vi "WLAN_be_EVM_SA.vi"(5 "Function":T1, 8 "error in":errorcluster, 11 "VISA IN":refnum<visa-resource-name>="IQGIG") -> (0 "error out":errorcluster, 1 "EVM":dbl format="%.0g", 2 "Power":dbl format="%#.3g", 3 "IDN":string)   [LabVIEW 2023, in "LitePoints.lvlib"]
uses:
  LitePoints.lvlib
  CTL/LitePoint_EVM_SA.ctl
  FTDI/JIO/CLC_JIO_FTDI.lvlib
panel:
  out "forREF_PW":string
  out "Response_EVM":string
  out "Response_PW":string
  out "VSA_Ref?":string
  out "VSA?":string
  out "Clean Buffer?":string
  # "IQgig-5G : TCPIP0::192.168.100.254::hislip0::INSTR"
  # "IQxel-MX : TCPIP0::192.168.100.253::hislip0::INSTR"
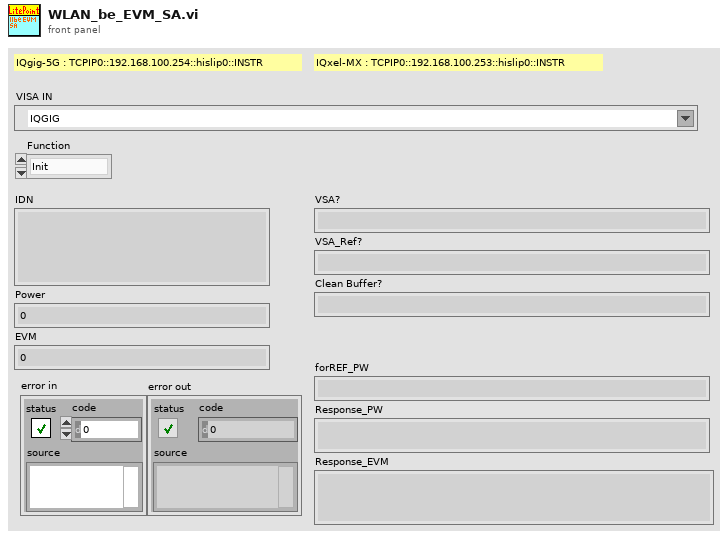
[diagram p1: front panel]
types:
  T1 = typedef "LitePoint_EVM_SA.ctl" = enum16{"Init", "Close", "set_SA", "get_EVM", "byPass", "getPower"}
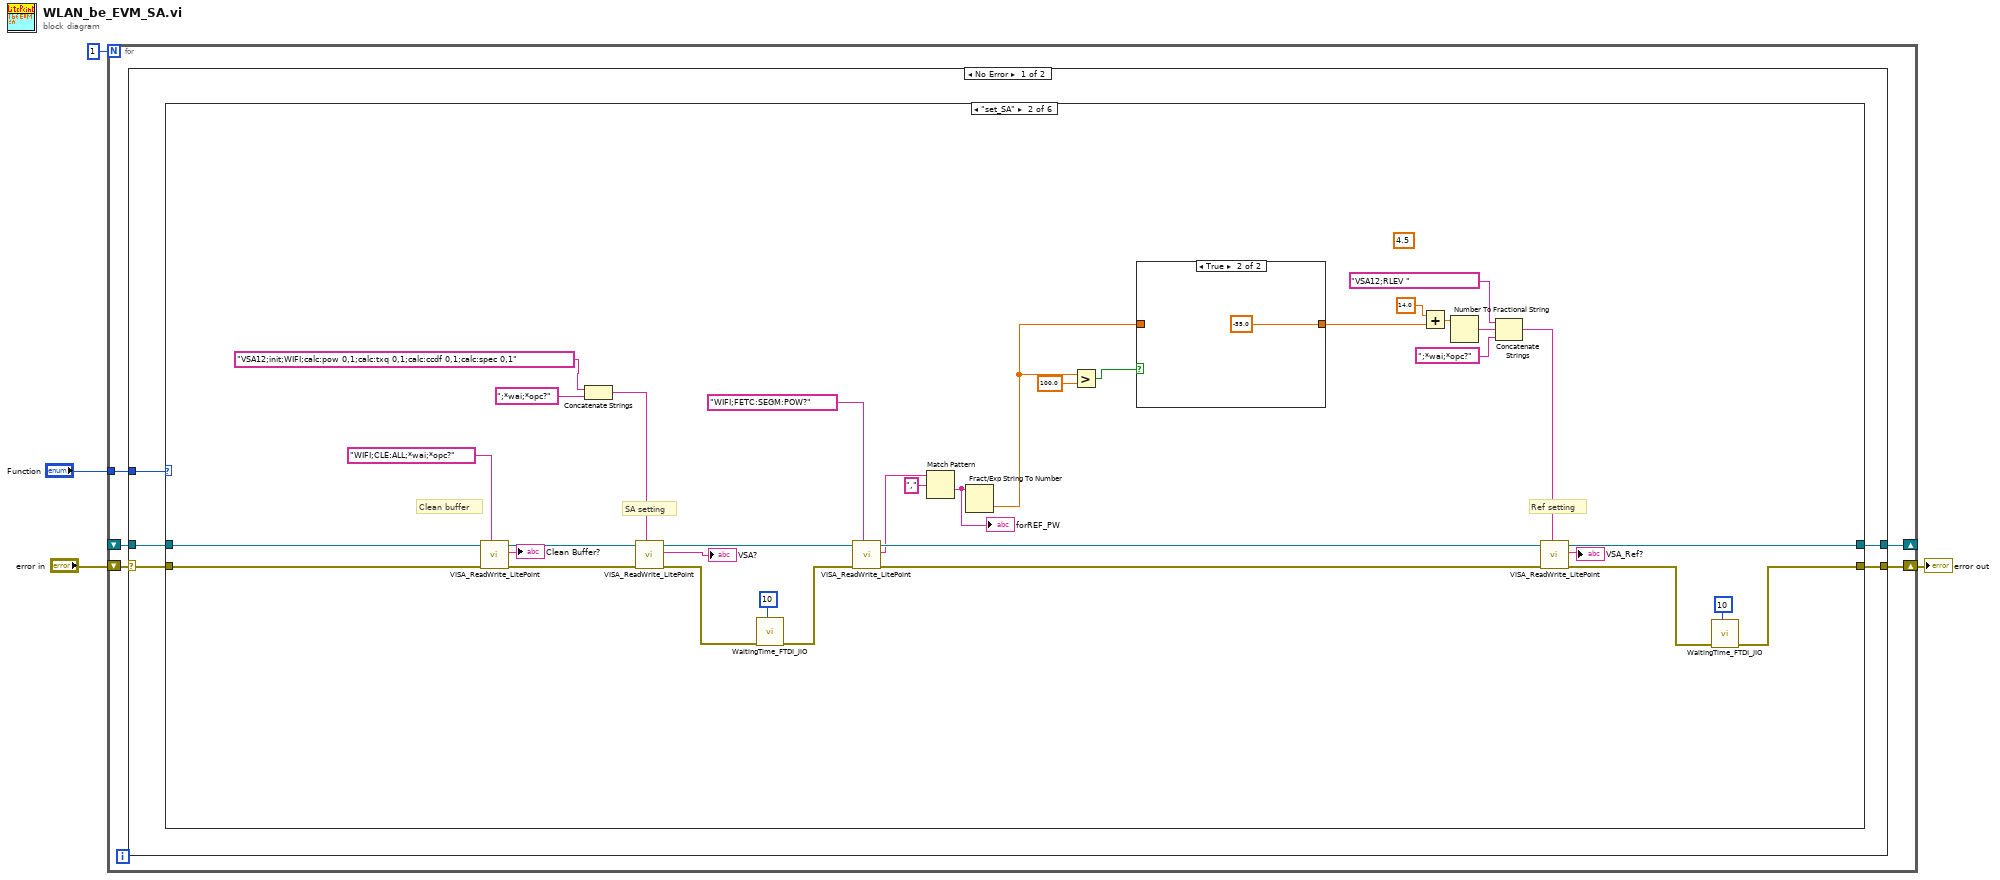
[diagram p0: block diagram]
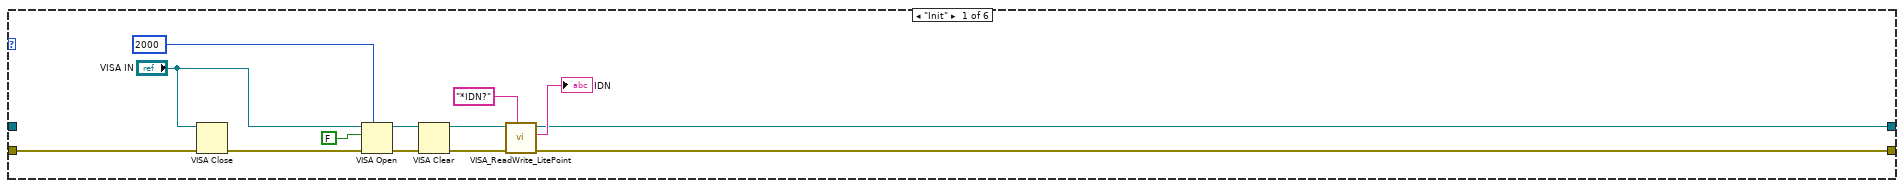
[diagram p2: hidden frame]
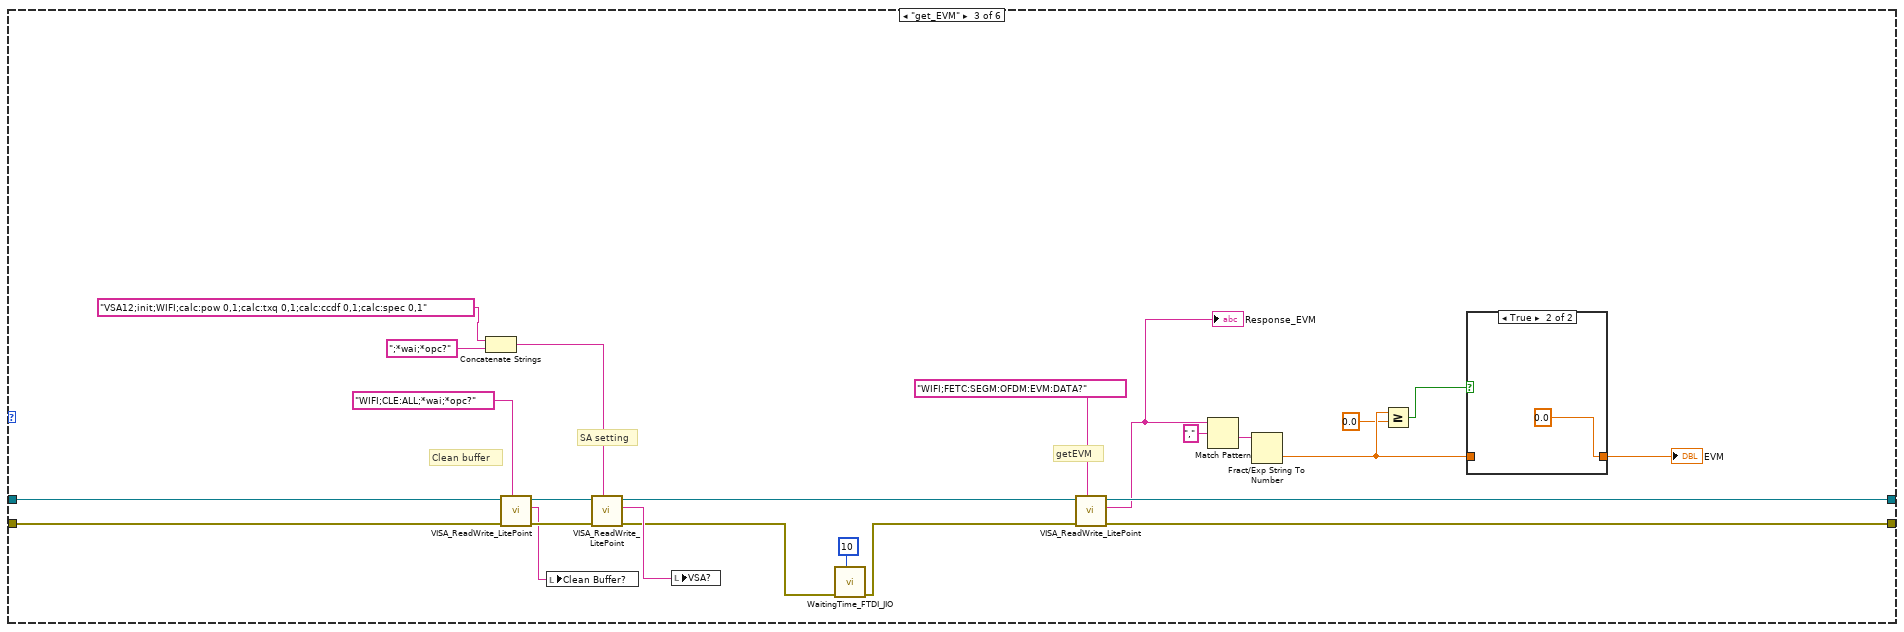
[diagram p4: hidden frame]
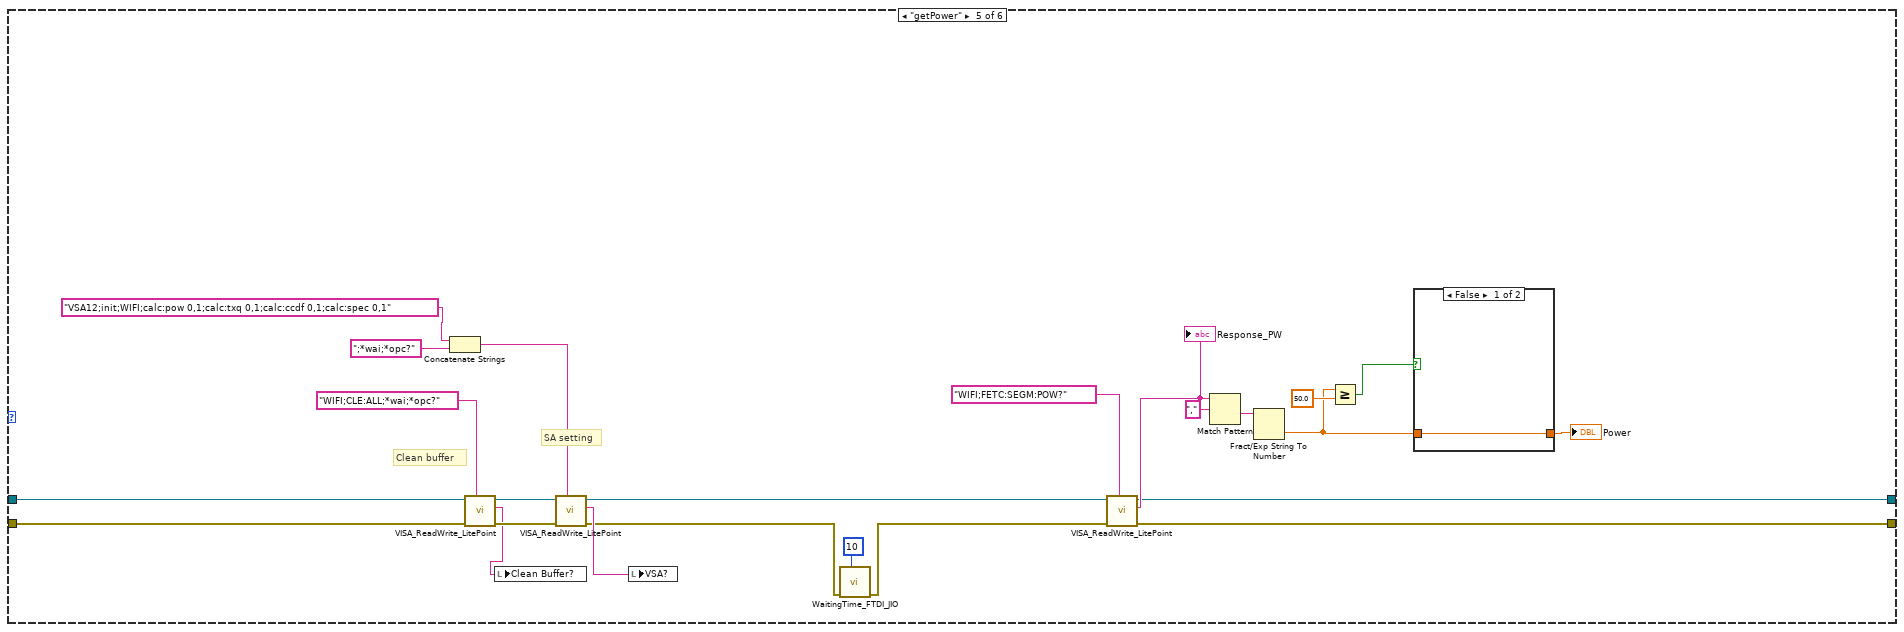
[diagram p7: hidden frame]
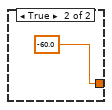
[diagram p8: hidden frame]
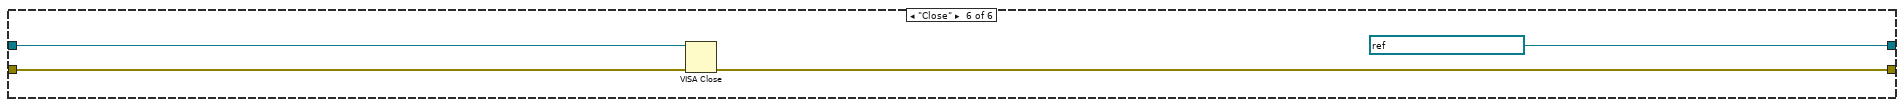
[diagram p9: hidden frame]
diagram:
  n1 = for {
    N: 1 -> [_]
    tunnel: "Function" -> [w7]
    shift-right: [w8] -> w3
    shift-left: "error in" -> [w9]
    shift-right: [w5] -> _
    shift-left: _ -> [w6]
    n2 = case shown="No Error" w9 {
      selector: w9 -> [w13 w124]
      tunnel: [w12 w124] -> w8
      tunnel: w7 -> [w14 _]
      tunnel: w6 -> [w11 w123]
      tunnel: [w10 w123] -> w5
      frame No Error {
        n3 = case shown="\"set_SA\"" w14 {
          tunnel: [w22 w33 w87 w92 w116 w122] -> w12
          tunnel: w13 -> [w17 w62 w72 w92 w105 w121]
          tunnel: w11 -> [_ w61 w71 w91 w102 w120]
          tunnel: [w18 w50 w86 w91 w111 refnum<visa-resource-name> refnum ("VISA out")] -> w10
          frame "Init" {
            n4 = VISA Close(VISA resource name="VISA IN", error in (no error)=w17) -> (error out=w16:errorcluster)
            n5 = VISA Open(timeout (0)=u32 2000 ("VISA Open timeout (0)"), duplicate session (F)=FALSE, error in (no error)=w16, VISA resource name="VISA IN") -> (VISA resource name=w24:refnum<visa-resource-name>, error out=w25:errorcluster)  [unwired: 1 in]
            n6 = VISA Clear(VISA resource name=w24, error in (no error)=w25) -> (VISA resource name out=w21:refnum<visa-resource-name>, error out=w23:errorcluster)
            n7 = call "VISA_ReadWrite_LitePoint.vi"("VISA_CMD"="*IDN?", "error in"=w23, "VISA in"=w21) -> ("error out"=w22:errorcluster, "Response"=→"IDN":string, "VISA out"=w18:refnum<visa-resource-name>)  [unwired: 6 in]
          }
          frame "set_SA" {
            (unwired) 4.5 ("x")
            # "Ref setting"
            # "SA setting"
            # "Clean buffer"
            n8 = call "VISA_ReadWrite_LitePoint.vi"("VISA_CMD"="WIFI;CLE:ALL;*wai;*opc?" ("write buffer"), "error in"=w62, "VISA in"=w61) -> ("error out"=w55:errorcluster, "Response"=→"Clean Buffer?":string, "VISA out"=w56:refnum<visa-resource-name>)  [unwired: 6 in]
            n9 = Concatenate Strings("VSA12;init;WIFI;calc:pow 0,1;calc:txq 0,1;calc:ccdf 0,1;calc:spec 0,1" ("write buffer"), ";*wai;*opc?" ("write buffer")) -> (w57:string)
            n10 = call "VISA_ReadWrite_LitePoint.vi"("VISA_CMD"=w57, "error in"=w55, "VISA in"=w56) -> ("error out"=w30:errorcluster, "Response"=→"VSA?":string, "VISA out"=w44:refnum<visa-resource-name>)  [unwired: 6 in]
            n11 = call "WaitingTime_FTDI_JIO.vi"("Waiting Time(ms)"=u32 10, "error out"=w30) -> ("error out"=w29:errorcluster)  [unwired: 9 in]
            n12 = call "VISA_ReadWrite_LitePoint.vi"("VISA_CMD"="WIFI;FETC:SEGM:POW?" ("write buffer"), "error in"=w29, "VISA in"=w44) -> ("error out"=w45:errorcluster, "Response"=w39:string, "VISA out"=w43:refnum<visa-resource-name>)  [unwired: 6 in]
            n13 = Match Pattern(string=w39, regular expression=",") -> (after substring=w40:string)  [unwired: 1 in, 3 out]
            "forREF_PW" <- w40
            n14 = Fract/Exp String To Number(string=w40) -> (number=w37:dbl)  [unwired: 3 in, 1 out]
            n15 = Greater?(x=w37, y=100.0) -> (0:w35:bool)
            n16 = case shown="True" w35 {
              tunnel: w37 -> [w63 _]
              tunnel: [w63 -55.0 ("y")] -> w38
              frame False {
              }
              frame True {
              }
            }
            n17 = Add(x=14.0, y=w38) -> (x+y=w46:dbl)
            n18 = Number To Fractional String(number=w46) -> (F-format string=w51:string)  [unwired: 3 in]
            n19 = Concatenate Strings("VSA12;RLEV " ("write buffer"), w51, ";*wai;*opc?" ("write buffer")) -> (w49:string)
            n20 = call "VISA_ReadWrite_LitePoint.vi"("VISA_CMD"=w49, "error in"=w45, "VISA in"=w43) -> ("error out"=w34:errorcluster, "Response"=→"VSA_Ref?":string, "VISA out"=w50:refnum<visa-resource-name>)  [unwired: 6 in]
            n21 = call "WaitingTime_FTDI_JIO.vi"("Waiting Time(ms)"=u32 10, "error out"=w34) -> ("error out"=w33:errorcluster)  [unwired: 9 in]
          }
          frame "get_EVM" {
            # "SA setting"
            # "Clean buffer"
            # "getEVM"
            n22 = Concatenate Strings("VSA12;init;WIFI;calc:pow 0,1;calc:txq 0,1;calc:ccdf 0,1;calc:spec 0,1" ("write buffer"), ";*wai;*opc?" ("write buffer")) -> (w73:string)
            n23 = call "VISA_ReadWrite_LitePoint.vi"("VISA_CMD"="WIFI;CLE:ALL;*wai;*opc?" ("write buffer"), "error in"=w72, "VISA in"=w71) -> ("error out"=w74:errorcluster, "Response"=w69:string, "VISA out"=w75:refnum<visa-resource-name>)  [unwired: 6 in]
            n24 = local write "Clean Buffer?"(w69) -> ()
            n25 = call "VISA_ReadWrite_LitePoint.vi"("VISA_CMD"=w73, "error in"=w74, "VISA in"=w75) -> ("error out"=w66:errorcluster, "Response"=w68:string, "VISA out"=w70:refnum<visa-resource-name>)  [unwired: 6 in]
            n26 = local write "VSA?"(w68) -> ()
            n27 = call "WaitingTime_FTDI_JIO.vi"("Waiting Time(ms)"=u32 10, "error out"=w66) -> ("error out"=w65:errorcluster)  [unwired: 9 in]
            n28 = call "VISA_ReadWrite_LitePoint.vi"("VISA_CMD"="WIFI;FETC:SEGM:OFDM:EVM:DATA?" ("write buffer"), "error in"=w65, "VISA in"=w70) -> ("error out"=w87:errorcluster, "Response"=w84:string, "VISA out"=w86:refnum<visa-resource-name>)  [unwired: 6 in]
            "Response_EVM" <- w84
            n29 = Match Pattern(string=w84, regular expression=",") -> (after substring=w83:string)  [unwired: 1 in, 3 out]
            n30 = Fract/Exp String To Number(string=w83) -> (number=w81:dbl)  [unwired: 3 in, 1 out]
            n31 = Greater Or Equal?(x=w81, y=0.0) -> (x >= y?=w79:bool)
            n32 = case shown="True" w79 {
              tunnel: w81 -> [w89 _]
              tunnel: [w89 0.0] -> w82
              frame False {
              }
              frame True {
              }
            }
            "EVM" <- w82
          }
          frame "byPass", Default {
          }
          frame "getPower" {
            # "SA setting"
            # "Clean buffer"
            n33 = Concatenate Strings("VSA12;init;WIFI;calc:pow 0,1;calc:txq 0,1;calc:ccdf 0,1;calc:spec 0,1" ("write buffer"), ";*wai;*opc?" ("write buffer")) -> (w99:string)
            n34 = call "VISA_ReadWrite_LitePoint.vi"("VISA_CMD"="WIFI;CLE:ALL;*wai;*opc?" ("write buffer"), "error in"=w105, "VISA in"=w102) -> ("error out"=w100:errorcluster, "Response"=w98:string, "VISA out"=w101:refnum<visa-resource-name>)  [unwired: 6 in]
            n35 = local write "Clean Buffer?"(w98) -> ()
            n36 = call "VISA_ReadWrite_LitePoint.vi"("VISA_CMD"=w99, "error in"=w100, "VISA in"=w101) -> ("error out"=w94:errorcluster, "Response"=w97:string, "VISA out"=w96:refnum<visa-resource-name>)  [unwired: 6 in]
            n37 = local write "VSA?"(w97) -> ()
            n38 = call "WaitingTime_FTDI_JIO.vi"("Waiting Time(ms)"=u32 10, "error out"=w94) -> ("error out"=w93:errorcluster)  [unwired: 9 in]
            n39 = call "VISA_ReadWrite_LitePoint.vi"("VISA_CMD"="WIFI;FETC:SEGM:POW?" ("write buffer"), "error in"=w93, "VISA in"=w96) -> ("error out"=w116:errorcluster, "Response"=w112:string, "VISA out"=w111:refnum<visa-resource-name>)  [unwired: 6 in]
            "Response_PW" <- w112
            n40 = Match Pattern(string=w112, regular expression=",") -> (after substring=w113:string)  [unwired: 1 in, 3 out]
            n41 = Fract/Exp String To Number(string=w113) -> (number=w108:dbl)  [unwired: 3 in, 1 out]
            n42 = Greater Or Equal?(x=w108, y=50.0) -> (x >= y?=w109:bool)
            n43 = case shown="False" w109 {
              tunnel: w108 -> [w117 _]
              tunnel: [w117 -60.0] -> w107
              frame False {
              }
              frame True {
              }
            }
            "Power" <- w107
          }
          frame "Close" {
            n44 = VISA Close(VISA resource name=w120, error in (no error)=w121) -> (error out=w122:errorcluster)
          }
        }
      }
      frame Error {
      }
    }
  }
  "error out" <- w3
